vi "Destroy Notifiers.vi"(8 "error in (no error)":errorcluster, 11 "IED in":refnum<class "IED.lvclass">) -> (0 "error out":errorcluster, 3 "IED out":refnum<class "IED.lvclass">)   [LabVIEW 2015, in "IED Actor.lvlib" / "IED.lvclass"]
uses:
  IED.lvclass
  IED.lvclass/IED.ctl
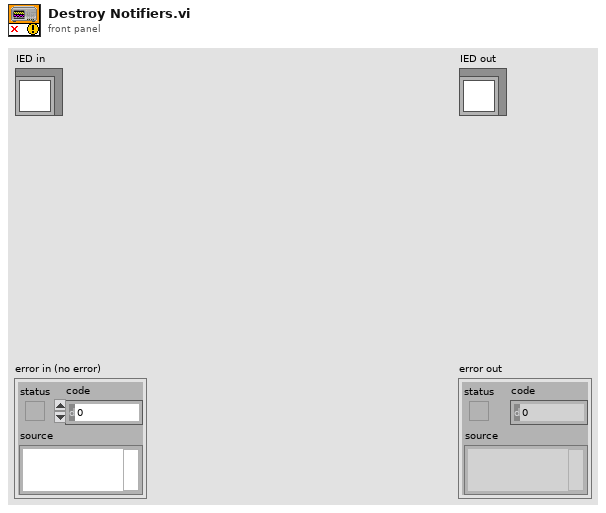
[diagram p1: front panel]
types:
  T1 = typedef "IED Actor.lvlib/IED.lvclass/Notifiers Cluster.ctl" = cluster{"stop":refnum<notifier>, "stop check":refnum<notifier>, "stop watchdog":refnum<notifier>, "IED stop":refnum<notifier>, "Island stop":refnum<notifier>, "Dog stop":refnum<notifier>}
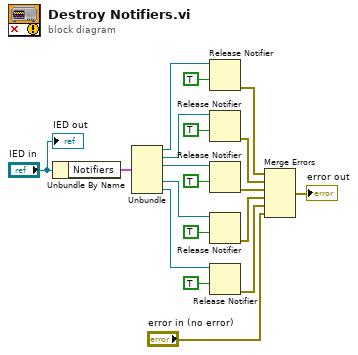
[diagram p0: block diagram]
diagram:
  n1 = Unbundle By Name("IED in") -> ("Notifiers"=w19:T1)
  n2 = Unbundle(w19) -> ("stop"=w15:refnum<notifier>, "stop check"=w14:refnum<notifier>, "stop watchdog"=w13:refnum<notifier>, "Island stop"=w12:refnum<notifier>, "Dog stop"=w11:refnum<notifier>)  [unwired: 1 out]
  n3 = Release Notifier(notifier=w15, force destroy? (F)=TRUE) -> (error out=w10:errorcluster)  [unwired: 1 in, 2 out]
  n4 = Release Notifier(notifier=w14, force destroy? (F)=TRUE) -> (error out=w9:errorcluster)  [unwired: 1 in, 2 out]
  n5 = Release Notifier(notifier=w13, force destroy? (F)=TRUE) -> (error out=w8:errorcluster)  [unwired: 1 in, 2 out]
  n6 = Release Notifier(notifier=w12, force destroy? (F)=TRUE) -> (error out=w7:errorcluster)  [unwired: 1 in, 2 out]
  n7 = Release Notifier(notifier=w11, force destroy? (F)=TRUE) -> (error out=w6:errorcluster)  [unwired: 1 in, 2 out]
  n8 = Merge Errors(w10, w9, w8, w7, w6, "error in (no error)") -> (→"error out":errorcluster)
  "IED out" <- "IED in"
